vi "Ball.vi"(6 "Ball Ref":cluster{refnum<vi>, "PaneColor":u32}[](array[cluster]), 8 "Cluster width":i32=200, 9 "Main Loop Iterations":i32=5, 10 "Ball Refs":refnum<vi>[](array[refnum]), 11 "Positions In":i32[](array[numeric])) -> (3 "Positions Out":i32[](array[numeric]))   [LabVIEW 2014]
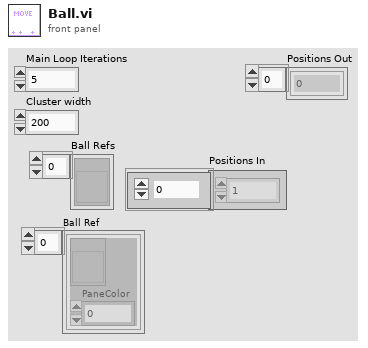
[diagram p1: front panel]
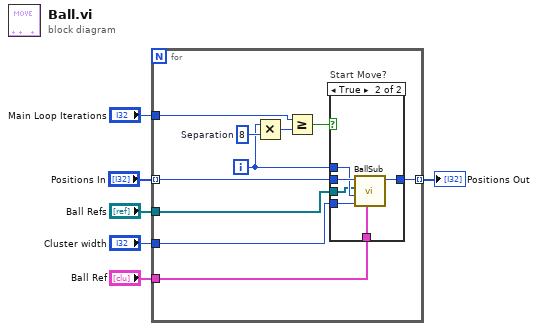
[diagram p0: block diagram]
diagram:
  n1 = for {
    tunnel: [w16] -> w6 mode=indexing
    tunnel: "Positions In" -> [w15] mode=indexing
    tunnel: "Ball Refs" -> [w13]
    tunnel: "Main Loop Iterations" -> [w10]
    tunnel: "Cluster width" -> [w8]
    tunnel: "Ball Ref" -> [w7]
    i -> [w12]
    w14 = 8  # Separation
    n2 = Multiply(x=w12, y=w14) -> (x*y=w11:i32)
    n3 = Greater Or Equal?(x=w10, y=w11) -> (x >= y?=w9:bool)
    n4 = case "Start Move?" shown="True" w9 {
      tunnel: [w17 w23] -> w16
      tunnel: w15 -> [w17 w22]
      tunnel: w12 -> [_ w21]
      tunnel: w13 -> [_ w20]
      tunnel: w8 -> [_ w19]
      tunnel: w7 -> [_ w18]
      frame False {
      }
      frame True {
        n5 = call "BallSub.vi"("Ball Ref"=w18, "Cluster width"=w19, "Ball Nr"=w21, "Ball Refs"=w20, "Position In"=w22) -> ("Position out"=w23:i32)  [unwired: 6 out]
      }
    }
  }
  "Positions Out" <- w6
